vi "Amplifier Output.vi"(0 "Filter":refnum<vi>, 2 "Filtered":T2, 5 "Filter Led Indicator":refnum<vi>, 11 "error in":errorcluster, 12 "Signal Acquisition":T3 {"Scale Type" items=["Volts"=10348, "Custom Scale"=10065]; "Sample Mode" items=["Finite Samples"=10178, "Continuous Samples"=10123, "Hardware Timed Single Point"=12522]; "Terminal Configuration" items=["Default"=-1, "RSE"=10083, "Differential"=10106, "Pseudodifferential"=12529]}, 13 "IIR filter specifications":refnum<vi>, 14 "Exit":refnum<vi>) -> (15 "error out":errorcluster)   [LabVIEW 2012]
uses:
  <vilib>/DAQmx/read.llb/DAQmx Read (Analog Wfm 1Chan NSamp).vi
  <vilib>/DAQmx/create/channels.llb/DAQmx Create Channel (AI-Voltage-Basic).vi
  <vilib>/DAQmx/configure/timing.llb/DAQmx Timing (Sample Clock).vi
  <vilib>/measure/maspectr.llb/FFT Power Spectrum and PSD for 1 Chan.vi
  <vilib>/DAQmx/miscellaneous.llb/DAQmx Fill In Error Info.vi
  <vilib>/measure/macond.llb/IIR Filter for 1 Chan.vi
  <vilib>/measure/NI_MAPro.lvlib
panel:
  out "Exit":bool
  out "Filter Param":T1
  out "Filter":bool
  out "PSD":cluster{"f0":dbl, "df":dbl, "magnitude":dbl[]} {"magnitude" format="%.2p"; "f0" format="%0.2p"; "df" format="%0.2p"}
  out "signal out":waveform(dbl)
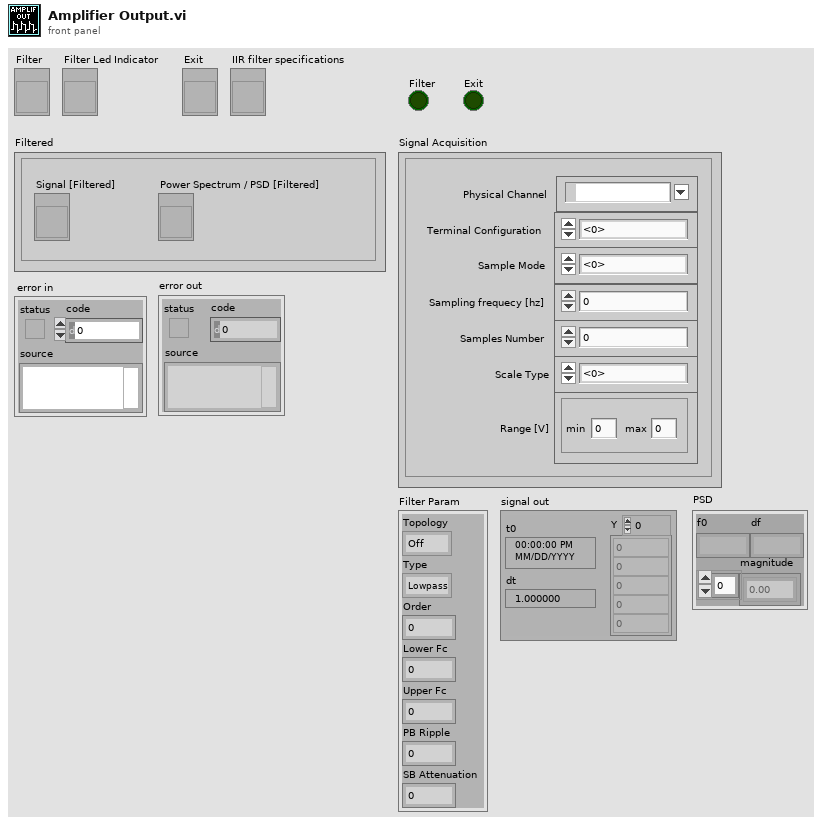
[diagram p1: front panel]
types:
  T1 = cluster{"Topology":enum16{"Off", "Butterworth", "Chebyshev", "Inverse Chebyshev", "Elliptic", "Bessel"}, "Type":enum16{"Lowpass", "Highpass", "Bandpass", "Bandstop"}, "Order":i32, "Lower Fc":dbl, "Upper Fc":dbl, "PB Ripple":dbl, "SB Attenuation":dbl}
  T2 = cluster{"Signal [Filtered]":refnum<vi>, "Power Spectrum / PSD [Filtered]":refnum<vi>}
  T3 = cluster{"Physical Channel":tag, "Terminal Configuration":i32, "Sample Mode":i32, "Scale Type":i32, "Range [V]":cluster{"max":dbl, "min":dbl}, "Sampling frequecy [hz]":dbl, "Samples Number":i32}
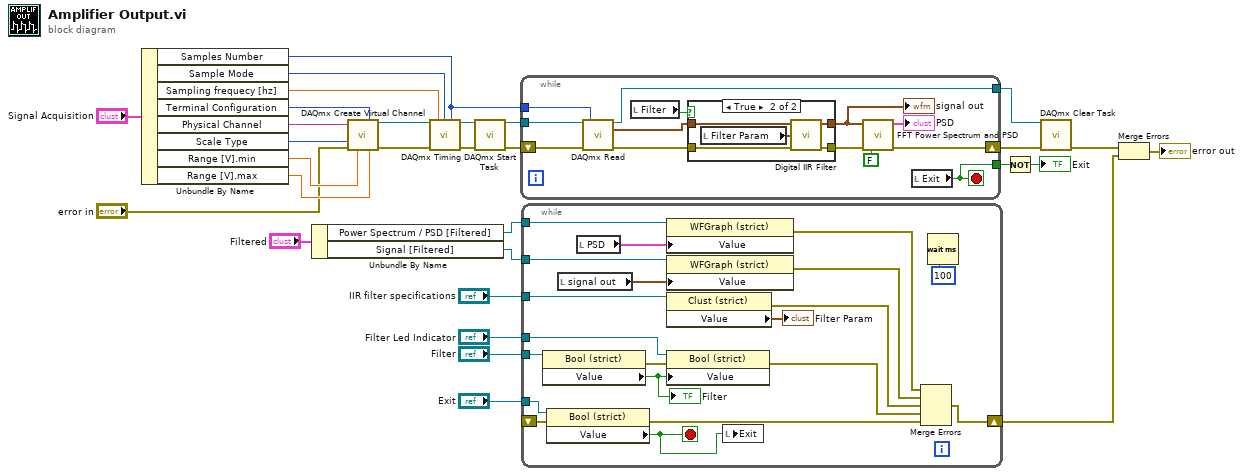
[diagram p0: block diagram]
diagram:
  n1 = Unbundle By Name("Signal Acquisition") -> ("Samples Number"=w23:i32, "Sample Mode"=w14:i32, "Sampling frequecy [hz]"=w22:dbl, "Terminal Configuration"=w21:i32, "Physical Channel"=w20:tag, "Scale Type"=w19:i32, "Range [V].min"=w18:dbl, "Range [V].max"=w17:dbl)
  n2 = Unbundle By Name("Filtered") -> ("Power Spectrum / PSD [Filtered]"=w6:refnum<vi>, "Signal [Filtered]"=w5:refnum<vi>)
  n3 = call-poly <vilib>:"DAQmx Create Virtual Channel.vi"("maximum value"=w17, "minimum value"=w18, "input terminal configuration"=w21, "physical channels"=w20, "units"=w19, "error in"="error in") -> ("task out"=w25:refnum<k21>, "error out"=w24:errorcluster)  [unwired: 8 in]
  n4 = call-poly <vilib>:"DAQmx Timing.vi"("task/channels in"=w25, "sample mode"=w14, "samples per channel"=w23, "rate"=w22, "error in"=w24) -> ("task out"=w27:refnum<k21>, "error out"=w26:errorcluster)  [unwired: 9 in]
  n5 = call <vilib>:"DAQmx Start Task.vi"("task/channels in"=w27, "error in"=w26) -> ("task out"=w29:refnum<k21>, "error out"=w28:errorcluster)  [unwired: 12 out]
  n6 = while {
    tunnel: w29 -> [w43]
    tunnel: w23 -> [w41]
    tunnel: [w38] -> w15
    shift-right: [w33] -> w30
    shift-left: w28 -> [w42]
    tunnel: [w31] -> w9
    stop <- w31 stop-if-true
    n7 = call-poly <vilib>:"DAQmx Read.vi"("task/channels in"=w43, "number of samples per channel"=w41, "error in"=w42) -> ("task out"=w38:refnum<k21>, "data"=w32:waveform(dbl), "error out"=w37:errorcluster)  [unwired: 10 in]
    n8 = local read "Filter"() -> (w34:bool)
    n9 = case shown="True" w34 {
      tunnel: w32 -> [w45 w50]
      tunnel: [w45 w49] -> w35
      tunnel: w37 -> [w44 w46]
      tunnel: [w44 w48] -> w39
      frame False {
      }
      frame True {
        n10 = local read "Filter Param"() -> (w47:T1)
        n11 = call-poly <vilib>:"Digital IIR Filter.vi"("IIR filter specifications"=w47, "error in (no error)"=w46, "signal in"=w50) -> ("error out"=w48:errorcluster, "signal out"=w49:waveform(dbl))  [unwired: 6 in, 1 out]
      }
    }
    "signal out" <- w35
    n12 = call-poly <vilib>:"FFT Power Spectrum and PSD.vi"("error in (no error)"=w39, "dB On (F)"=FALSE, "time signal"=w35) -> ("error out"=w33:errorcluster, "Power Spectrum / PSD"=→"PSD":cluster{"f0":dbl, "df":dbl, "magnitude":dbl[]})  [unwired: 5 in, 2 out]
    n13 = local read "Exit"() -> (w31:bool)
  }
  n14 = while {
    tunnel: "Filter Led Indicator" -> [w68]
    tunnel: "Filter" -> [w67]
    tunnel: "Exit" -> [w65]
    tunnel: w6 -> [w63]
    tunnel: w5 -> [w62]
    tunnel: "IIR filter specifications" -> [w60]
    shift-right: [w52] -> w2
    shift-left: _ -> [w53]
    stop <- w59 stop-if-true
    n15 = property class="Bool (strict)"(reference=w67) -> (error out=w58:errorcluster, "Value"=w66:bool)  [unwired: 1 in, 1 out]
    "Filter" <- w66
    n16 = property class="Bool (strict)"(reference=w65, error in=w53) -> (error out=w57:errorcluster, "Value"=w59:bool)  [unwired: 1 out]
    n17 = local read "signal out"() -> (w70:waveform(dbl))
    n18 = local read "PSD"() -> (w69:cluster{"f0":dbl, "df":dbl, "magnitude":dbl[]})
    n19 = property class="WFGraph (strict)"(reference=w63, "Value"=w69) -> (error out=w54:errorcluster)  [unwired: 1 in, 1 out]
    n20 = property class="WFGraph (strict)"(reference=w62, "Value"=w70) -> (error out=w51:errorcluster)  [unwired: 1 in, 1 out]
    n21 = property class="Clust (strict)"(reference=w60) -> (error out=w55:errorcluster, "Value"=→"Filter Param":T1)  [unwired: 1 in, 1 out]
    n22 = property class="Bool (strict)"(reference=w68, error in=w58, "Value"=w66) -> (error out=w56:errorcluster)  [unwired: 1 out]
    n23 = local write "Exit"(w59) -> ()
    n24 = Merge Errors(w54, w51, w55, w56, w57) -> (w52:errorcluster)
    n25 = Wait (ms)(milliseconds to wait=u32 100) -> ()  [unwired: 1 out]
  }
  n26 = Not(x=w9) -> (.not. x?=→"Exit":bool)
  n27 = call <vilib>:"DAQmx Clear Task.vi"("task in"=w15, "error in"=w30) -> ("error out"=w3:errorcluster)  [unwired: 13 in]
  n28 = Merge Errors(w3, w2) -> (→"error out":errorcluster)
